vi "UpdateReferenceObject.vi"(0 "reference in":refnum<class "G#RemoteProxy.lvclass">, 5 "error in (no error)":errorcluster) -> (14 "reference out":refnum<class "G#RemoteProxy.lvclass">, 19 "error out":errorcluster)   [LabVIEW 2017, in "G#RemoteProxy.lvclass"]
doc: "Update reference object to be a valid object."
uses:
  <vilib>/addons/_AddQ/G#Debugger/G#RemoteProxy/G#RemoteProxy.lvclass
  C:/Program Files (x86)/National Instruments/LabVIEW 2017/vi.lib/addons/_AddQ/G#Object/G#Object.lvclass
  <vilib>/addons/_AddQ/G#Object/G#Object.lvclass
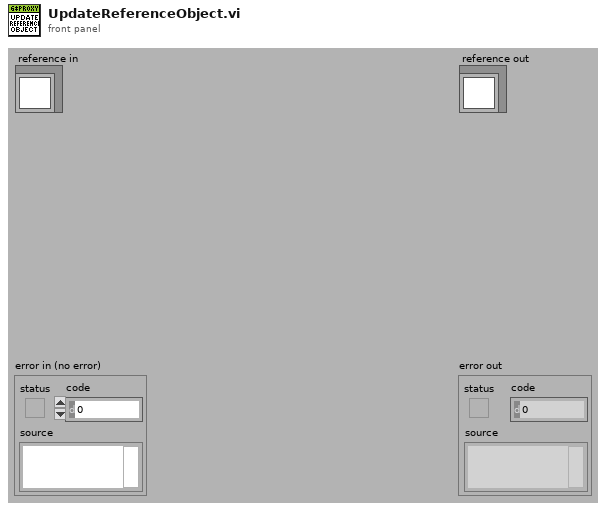
[diagram p1: front panel]
types:
  T1 = typedef "G#RemoteProxy.lvclass/ObjectAttributesProxy.ctl" = cluster{"class hierarchy":T2[], "class name":string, "lvlib hierarchy":string[], "full class name":string, "id":u32, "owner":string, "RemoteRef":refnum<class "G#Object.lvclass">, "object name":string, "attributes":variant[], "connection ID":refnum<k5>, "address":u32, "occurrence":refnum<k4>, "ProxyClassRef":refnum<class "G#RemoteProxy.lvclass">, "InMemory?":bool, "ToString":string}
  T2 = typedef "G#Object.lvclass/G#Object_ClassHierarchy.ctl" = cluster{"ClassName":string, "FullClassName":string, "ClassPath":path, "IsLeaf":bool}
  T3 = cluster{"full class name":string, "G#Object.lvclass":refnum<class "G#Object.lvclass">}
  T4 = cluster{"full class name":string, "G#Object.lvclass":refnum<class "G#Object.lvclass">}[]
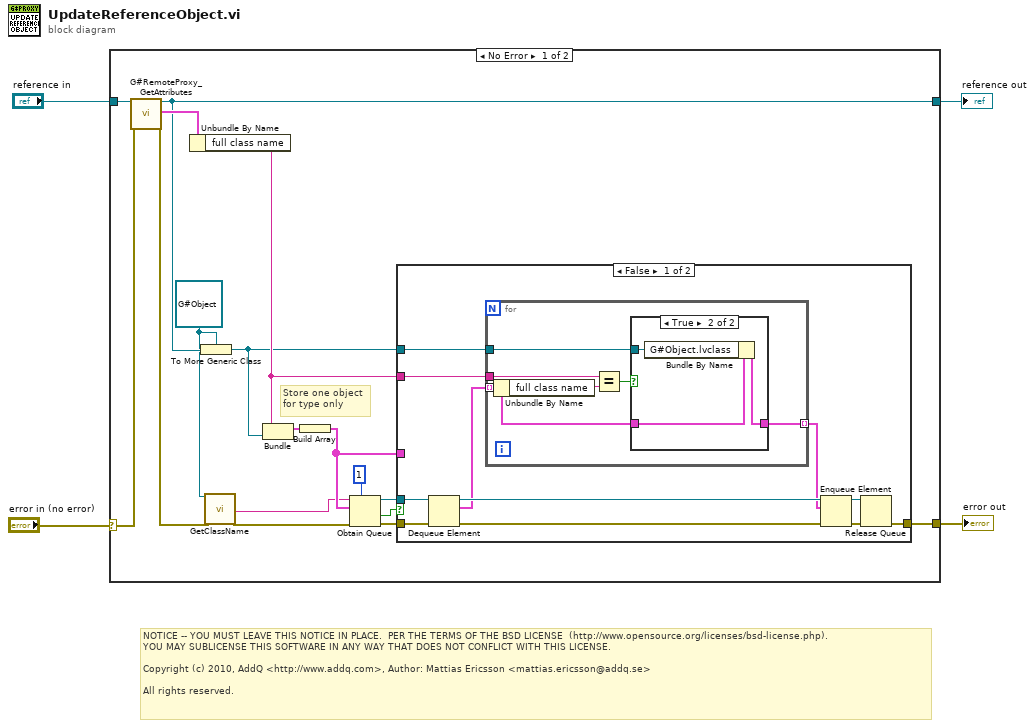
[diagram p0: block diagram]
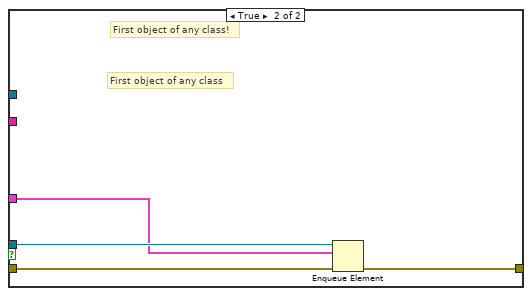
[diagram p3: hidden frame]
diagram:
  # "NOTICE -- YOU MUST LEAVE THIS NOTICE IN PLACE.  PER THE TERMS OF THE BSD LICENSE  (http://www.opensource.org/licenses/bsd-license.php).\nYOU MAY SUBLICENSE THIS SOFTWARE IN ANY WAY THAT DOES NOT CONFLICT WITH THIS LICENSE.\n\nCopyright (c) 2010, AddQ <http://www.addq.com>, Author: Mattias Ericsson <mattias.ericsson@addq.se>\n\nAll rights reserved."
  n1 = case shown="No Error" "error in (no error)" {
    selector: "error in (no error)" -> [w21 w48]
    tunnel: [w14 w48] -> w3
    tunnel: [w12 w47] -> w1
    tunnel: "reference in" -> [w19 w47]
    frame No Error {
      w6 = refnum<class "G#Object.lvclass"> refnum ("G#Object.lvclass")
      # "Store one object\nfor type only"
      n2 = call <vilib>:"G#RemoteProxy_GetAttributes.vi"("reference in"=w19, "error in (no error)"=w21) -> ("reference out"=w12:refnum<class "G#RemoteProxy.lvclass">, "attributes"=w20:T1, "error out"=w8:errorcluster)  [unwired: 14 in, 1 out]
      n3 = Unbundle By Name(w20) -> ("full class name"=w10:string)
      n4 = To More Generic Class(target class=w6, reference=w12) -> (generic class reference=w9:refnum<class "G#Object.lvclass">)
      n5 = call-dynamic "GetClassName.vi"("reference in"=w6, "error in (no error)"=w8) -> ("full class name"=w5:string, "error out"=w7:errorcluster)  [unwired: 13 in, 3 out]
      n6 = Bundle("full class name"=w10, "G#Object.lvclass"=w9) -> (w18:T3)  [unwired: 1 in]
      n7 = Build Array(w18) -> (w13:T4)
      n8 = Obtain Queue(max queue size (-1, unlimited)=1, name (unnamed)=w5, element data type=w13, error in (no error)=w7) -> (queue out=w16:refnum<queue>, created new?=w15:bool, error out=w17:errorcluster)  [unwired: 1 in]
      n9 = case shown="False" w15 {
        tunnel: w17 -> [w32 w46]
        tunnel: [w26 w45] -> w14
        tunnel: w16 -> [w31 w44]
        tunnel: w13 -> [_ w43]
        tunnel: w10 -> [w24 _]
        tunnel: w9 -> [w23 _]
        frame False {
          n10 = Dequeue Element(queue=w31, error in (no error)=w32) -> (queue out=w30:refnum<queue>, element=w25:T4, error out=w27:errorcluster)  [unwired: 1 in, 1 out]
          n11 = for {
            tunnel: w25 -> [w35] mode=indexing
            tunnel: w24 -> [w37]
            tunnel: w23 -> [w34]
            tunnel: [w33] -> w22 mode=indexing
            n12 = Unbundle By Name(w35) -> ("full class name"=w38:string)
            n13 = Equal?(x=w37, y=w38) -> (x = y?=w36:bool)
            n14 = case shown="True" w36 {
              tunnel: w35 -> [w39 w42]
              tunnel: w34 -> [_ w41]
              tunnel: [w39 w40] -> w33
              frame False {
              }
              frame True {
                n15 = Bundle By Name(cluster=w42, "G#Object.lvclass"=w41) -> (w40:T3)
              }
            }
          }
          n16 = Enqueue Element(queue=w30, element=w22, error in (no error)=w27) -> (queue out=w28:refnum<queue>, error out=w29:errorcluster)  [unwired: 1 in, 1 out]
          n17 = Release Queue(queue=w28, error in (no error)=w29) -> (error out=w26:errorcluster)  [unwired: 1 in, 2 out]
        }
        frame True {
          # "First object of any class"
          # "First object of any class!"
          n18 = Enqueue Element(queue=w44, element=w43, error in (no error)=w46) -> (error out=w45:errorcluster)  [unwired: 1 in, 2 out]
        }
      }
    }
    frame Error {
    }
  }
  "error out" <- w3
  "reference out" <- w1
